vi "Function Mode.vi"(5 "Enable to Query":bool, 7 "Enable to Setup":bool, 8 "error in":errorcluster, 10 "Function Mode":u8(ring) items=["AUTO"=1, "MANU"=0], 11 "VISA resource name":refnum<visa-resource-name>) -> (0 "error out":errorcluster, 2 "Query the Function Mode":string, 3 "VISA resource name out":refnum<visa-resource-name>)   [LabVIEW 2011, in "GPT-9000.lvlib"]
uses:
  <instrlib>/GPT-9000/GPT-9000.lvlib
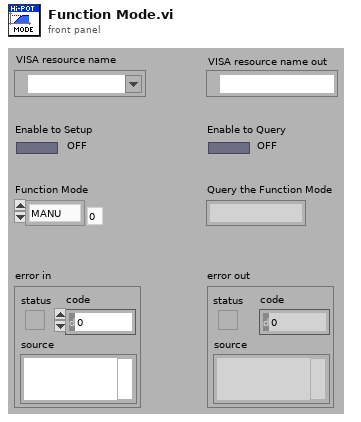
[diagram p1: front panel]
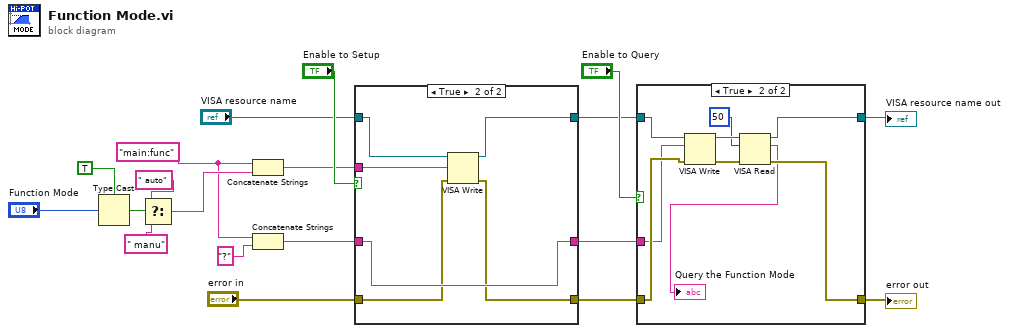
[diagram p0: block diagram]
diagram:
  w14 = "main:func"
  n1 = Type Cast(type=TRUE, x="Function Mode") -> (*(type *) &x=w16:bool)
  n2 = Select(t=" auto", s=w16, f=" manu") -> (s? t:f=w19:string)
  n3 = Concatenate Strings(w14, w19) -> (w9:string)
  n4 = Concatenate Strings(w14, "?" ("string")) -> (w8:string)
  n5 = case shown="True" "Enable to Setup" {
    tunnel: "VISA resource name" -> [w22 w27]
    tunnel: "error in" -> [w21 w26]
    tunnel: [w22 w25] -> w5
    tunnel: [w21 w24] -> w4
    tunnel: w9 -> [_ w23]
    tunnel: w8 -> [w20 w28]
    tunnel: [w20 w28] -> w3
    frame False {
    }
    frame True {
      n6 = VISA Write(VISA resource name=w27, write buffer=w23, error in (no error)=w26) -> (VISA resource name out=w25:refnum<visa-resource-name>, error out=w24:errorcluster)  [unwired: 1 out]
    }
  }
  n7 = case shown="True" "Enable to Query" {
    tunnel: w5 -> [w30 w39]
    tunnel: [w30 w34] -> w2
    tunnel: w4 -> [w29 w38]
    tunnel: [w29 w33] -> w1
    tunnel: w3 -> [_ w37]
    frame False {
    }
    frame True {
      n8 = VISA Write(VISA resource name=w39, write buffer=w37, error in (no error)=w38) -> (VISA resource name out=w35:refnum<visa-resource-name>, error out=w36:errorcluster)  [unwired: 1 out]
      n9 = VISA Read(VISA resource name=w35, byte count=u32 50, error in (no error)=w36) -> (VISA resource name out=w34:refnum<visa-resource-name>, read buffer=→"Query the Function Mode":string, error out=w33:errorcluster)  [unwired: 1 out]
    }
  }
  "VISA resource name out" <- w2
  "error out" <- w1
